vi "readTableAsString.vi"(8 "error in (no error)":errorcluster, 11 "Document in":refnum<class "Document.lvclass">) -> (0 "error out":errorcluster, 2 "Table":string[][](array[string]), 3 "Document out":refnum<class "Document.lvclass">)   [LabVIEW 2017, in "LabVIEW NPOI.lvlib" / "Document.lvclass"]
doc: "Protected dynamic dispatch method to append the wire <b>Table</b> as 2D array of strings to the <b>Document</b> as a table."
uses:
  Document.lvclass
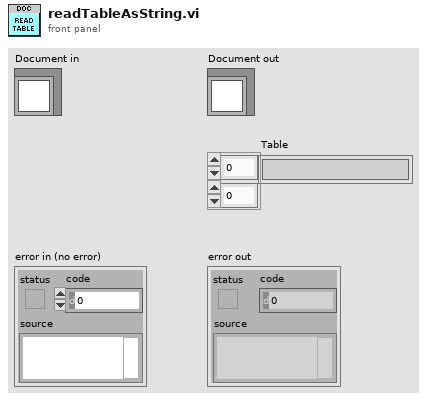
[diagram p1: front panel]
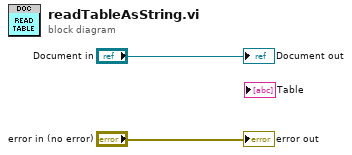
[diagram p0: block diagram]
diagram:
  "error out" <- "error in (no error)"
  "Document out" <- "Document in"
